vi "Configure Active DUT Control IP Endpoint.vi"(8 "error in (no error)":errorcluster, 10 "IP Endpoint (\"localhost:5000\")":string="localhost:5000", 11 "VISA resource name":refnum<visa-resource-name>) -> (0 "error out":errorcluster, 3 "VISA resource name out":refnum<visa-resource-name>)   [LabVIEW 2020, in "Rohde&Schwarz CMXP Base.lvlib"]
doc: "Specifies an IP address and port for communication with the external automation application.\n\nAttribute:\nRSCMXPBASE_ATTR_ACTIVE_DUT_CONTROL_IP_ENDPOINT\n\nRemote-control command:\n[CONFigure:]DUT:CONTrol:AUTO:EXTernal:IPADdr"
uses:
  <instrlib>/Rohde&Schwarz CMXP Base/Rohde&Schwarz CMXP Base.lvlib
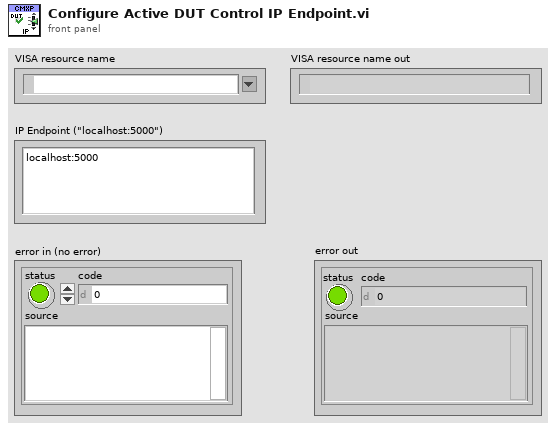
[diagram p1: front panel]
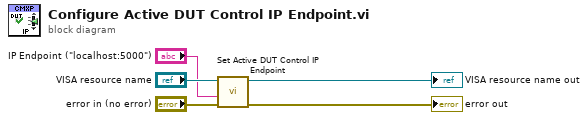
[diagram p0: block diagram]
diagram:
  n1 = call "Set Active DUT Control IP Endpoint"("error in (no error)"="error in (no error)", "Active DUT Control IP Endpoint ()"="IP Endpoint (\"localhost:5000\")", "instrument handle"="VISA resource name") -> ("error out"=→"error out":errorcluster, "instrument handle out"=→"VISA resource name out":refnum<visa-resource-name>)  [unwired: 7 in]
